vi "SetE Cal Port Map.vi"(8 "error in (no error)":errorcluster {"code" format="%.0x"}, 9 "PortMaping":string, 10 "Module":string, 11 "instrument handle":refnum<k15>) -> (0 "error out":errorcluster {"code" format="%.0x"}, 3 "instrument handle out":refnum<k15>)   [LabVIEW 2014, in "Agilent NA.lvlib"]
doc: "This command specifies the port mapping (which ports of the module are connected to which ports of the PNA) prior to performing ECal calibrations."
uses:
  Agilent NA.lvlib
  AgNA.dll
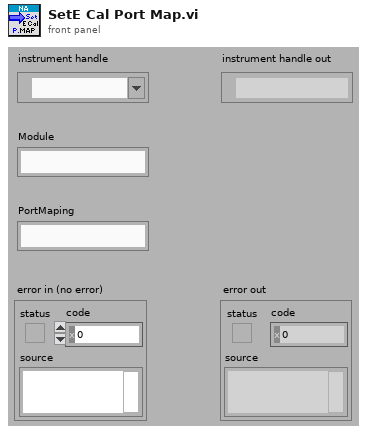
[diagram p1: front panel]
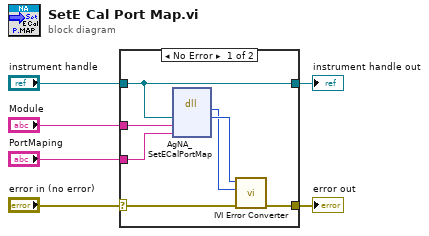
[diagram p0: block diagram]
diagram:
  n1 = case shown="No Error" "error in (no error)" {
    selector: "error in (no error)" -> [w11 w15]
    tunnel: [w10 w15] -> w6
    tunnel: "Module" -> [w9 _]
    tunnel: "PortMaping" -> [w8 _]
    tunnel: "instrument handle" -> [w7 w14]
    tunnel: [w7 w14] -> w1
    frame No Error {
      n2 = dll-call lib="AgNA**.dll" fn="AgNA_SetECalPortMap"("Vi"=w7, "Module"=w9, "PortMaping"=w8) -> (w12:i32, "Vi"=w13:u32)  [unwired: 5 in, 2 out]
      n3 = call "IVI Error Converter.vi"("error in (no error)"=w11, "IVI error code (0)"=w12, "instrument handle"=w13) -> ("error out"=w10:errorcluster)  [unwired: 7 in, 1 out]
    }
    frame Error {
    }
  }
  "error out" <- w6
  "instrument handle out" <- w1
